vi "Parse 14.vi"(11 "String":string) -> (3 "Puzzle":T1)   [LabVIEW 2020]
uses:
  Puzzle 14.ctl
  <vilib>/regexp/Match Regular Expression.xnode
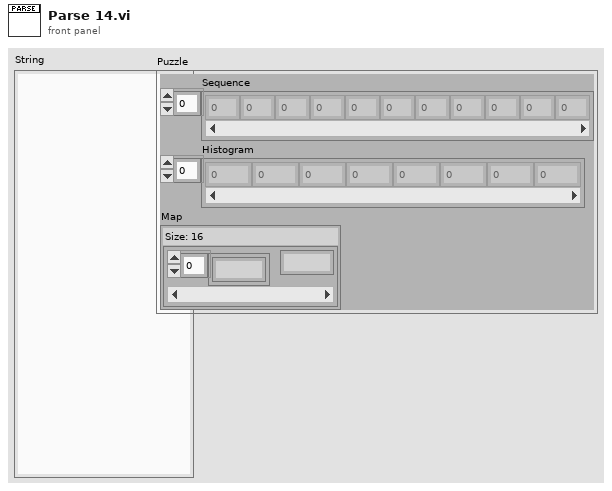
[diagram p1: front panel]
types:
  T1 = typedef "Puzzle 14.ctl" = cluster{"Sequence":u8[], "Histogram":u64[], "Map":map{u8[], u8}}
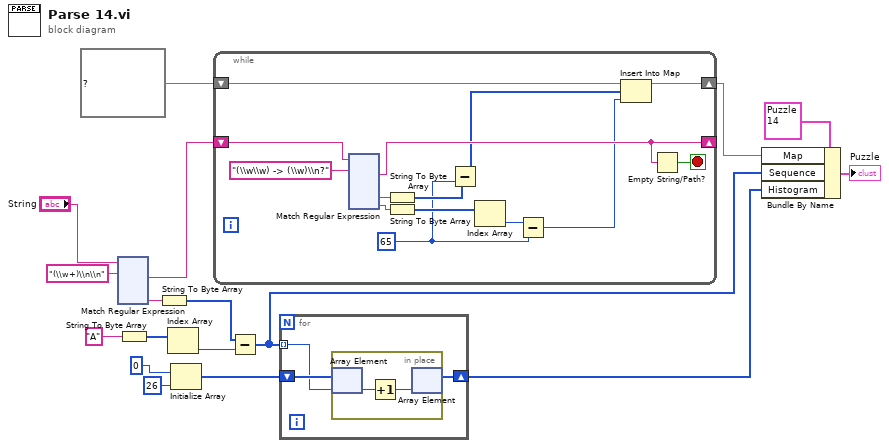
[diagram p0: block diagram]
diagram:
  n1 = xnode "Match Regular Expression"("input string"="String", "regular expression"="(\\w+)\\n\\n") -> ("after match"=w3:string, "submatch 1"=w15:string)  [unwired: 4 in, 4 out]
  n2 = String To Byte Array(string="A") -> (unsigned byte array=w13:u8[])
  n3 = String To Byte Array(string=w15) -> (unsigned byte array=w6:u8[])
  n4 = Index Array(array=w13) -> (element=w12:u8)  [unwired: 1 in]
  n5 = Initialize Array(u64 0, 26 ("dimension size")) -> (w9:u64[])
  n6 = while {
    shift-right: [w21] -> w4
    shift-left: map{u8[], u8} {} ("Map") -> [w24]
    shift-right: [w27] -> _
    shift-left: w3 -> [w31]
    stop <- w26 stop-if-true
    w18 = u8 65 ("y")
    n7 = xnode "Match Regular Expression"("input string"=w31, "regular expression"="(\\w\\w) -> (\\w)\\n?") -> ("after match"=w27:string, "submatch 1"=w29:string, "submatch 2"=w28:string)  [unwired: 4 in, 4 out]
    n8 = String To Byte Array(string=w29) -> (unsigned byte array=w23:u8[])
    n9 = String To Byte Array(string=w28) -> (unsigned byte array=w25:u8[])
    n10 = Subtract(x=w23, y=w18) -> (x-y=w19:u8[])
    n11 = Index Array(array=w25) -> (element=w22:u8)  [unwired: 1 in]
    n12 = Subtract(x=w22, y=w18) -> (x-y=w20:u8)
    n13 = Insert Into Map(map in=w24, key=w19, value=w20) -> (map out=w21:map{u8[], u8})  [unwired: 2 out]
    n14 = Empty String/Path?(string/path=w27) -> (empty?=w26:bool)
  }
  n15 = Subtract(x=w6, y=w12) -> (x-y=w1:u8[])
  n16 = for {
    tunnel: w1 -> [w150] mode=indexing
    shift-right: [w149] -> w7
    shift-left: w9 -> [w151]
    n17 = in-place {
      n18 = in-place-array #1(w151, w150) -> (w153:u64)
      n19 = Increment(x=w153) -> (x+1=w152:u64)
      n20 = in-place-array #1(w152) -> (w149:u64[])  [unwired: 1 out]
    }
  }
  n21 = Bundle By Name(cluster=T1 {"Sequence"=[], "Histogram"=[], "Map"={}} ("Puzzle"), "Map"=w4, "Sequence"=w1, "Histogram"=w7) -> (→"Puzzle":T1)
